vi "DS360 Set Offset.vi"(8 "error in (no error)":T1, 10 "DC offset":ext, 11 "GPIB address":string) -> (0 "error out":T1, 3 "address out":string)   [LabVIEW 2025, in "MyDS360.lvlib"]
uses:
  MyDS360.lvlib
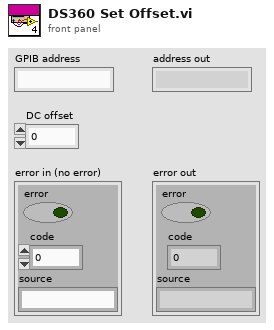
[diagram p1: front panel]
types:
  T1 = cluster{"error":bool, "code":i32, "source":string}
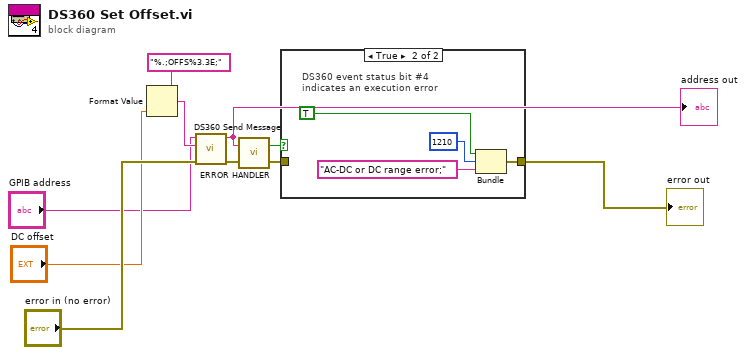
[diagram p0: block diagram]
diagram:
  n1 = Format Value(format string="%.;OFFS%3.3E;", value (0)="DC offset") -> (output string=w4:string)  [unwired: 1 in]
  n2 = call "DS360 Send Message.vi"("address string"="GPIB address", "write buffer"=w4, "error in"="error in (no error)") -> ("address out"=w8:string, "error out"=w9:T1)  [unwired: 3 in, 2 out]
  "address out" <- w8
  n3 = call "ERROR HANDLER.vi"("error in"=w9, "GPIB address"=w8) -> ("error out"=w7:T1, "error found"=w6:bool)
  n4 = case shown="True" w6 {
    tunnel: w7 -> [w11 _]
    tunnel: [w11 w12] -> w10
    frame False {
    }
    frame True {
      # "DS360 event status bit #4\nindicates an execution error"
      n5 = Bundle(TRUE, 1210, "AC-DC or DC range error;") -> (w12:errorcluster)  [unwired: 1 in]
    }
  }
  "error out" <- w10
